vi "checkSamplingRates.vi"(8 "error in (no error)":errorcluster, 11 "Available Sigals in":refnum<class "ISignal.lvclass">[](array[class])) -> (0 "error out":errorcluster, 1 "SampleRate":dbl, 2 "Boolean":bool, 3 "Array":refnum<class "ISignal.lvclass">[](array[class]))   [LabVIEW 2022 SP3, in "MultiReader.lvlib"]
uses:
  <instrlib>/openDAQ/Examples/MultiReader/MultiReader.lvlib
  <instrlib>/openDAQ/Public/Classes/ISignal/ISignal.lvclass
  <instrlib>/openDAQ/Public/Classes/IBaseObject/Polymorphic/queryInterface/queryNumberInterface.vi
  <instrlib>/openDAQ/Public/Classes/IDataDescriptor/IDataDescriptor.lvclass
  <instrlib>/openDAQ/Public/Classes/IDataRule/IDataRule.lvclass
  <instrlib>/openDAQ/Public/Classes/daqCoreTypes/IRatio/IRatio.lvclass
  <instrlib>/openDAQ/Public/Classes/daqCoreTypes/IDict/IDict.lvclass
  <instrlib>/openDAQ/Public/Classes/IBaseObject/IBaseObject.lvclass
  <instrlib>/openDAQ/Public/Classes/daqCoreTypes/INumber/INumber.lvclass
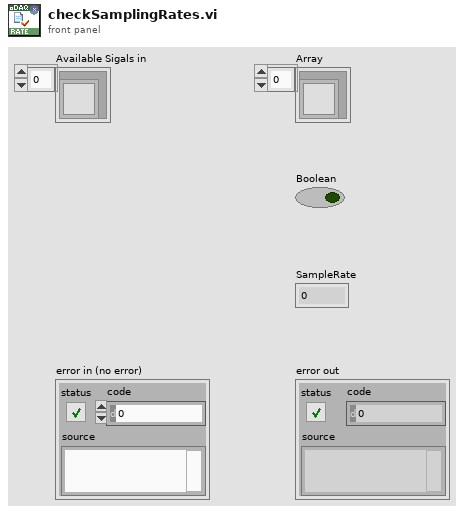
[diagram p1: front panel]
types:
  T1 = typedef "openDAQ.lvlib/IBaseObject.lvlib/IDataRule.lvlib/IDataRule.lvclass/DataRuleType.ctl" = u16
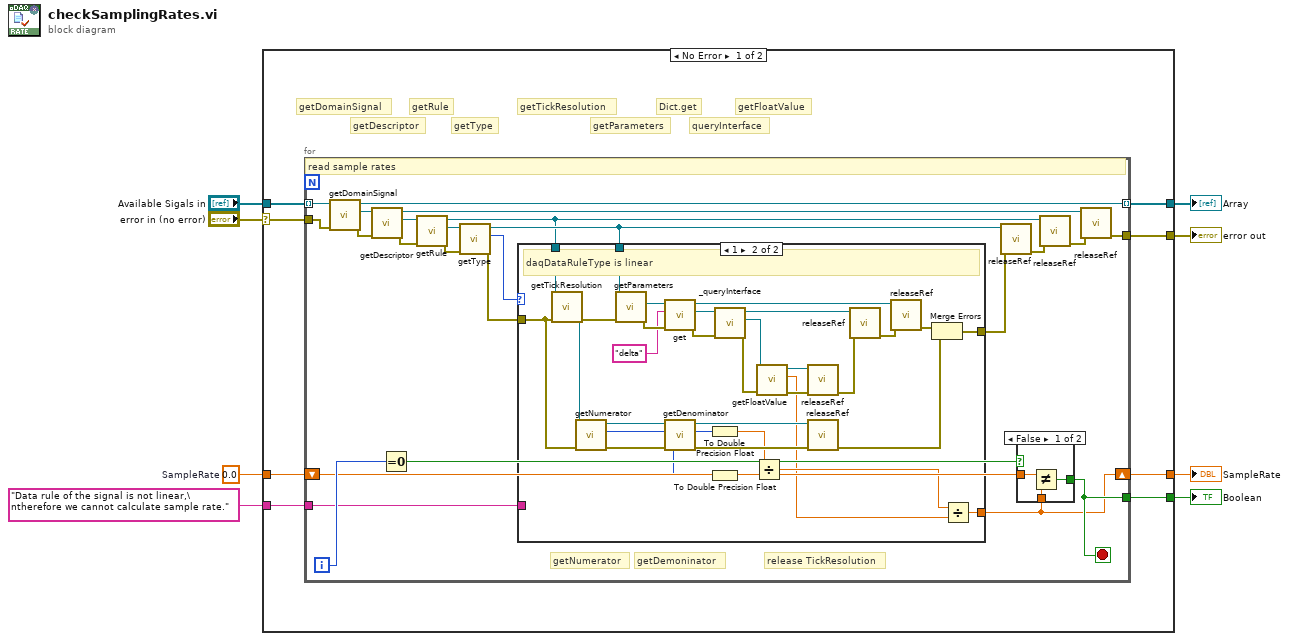
[diagram p0: block diagram]
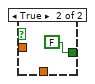
[diagram p2: hidden frame]
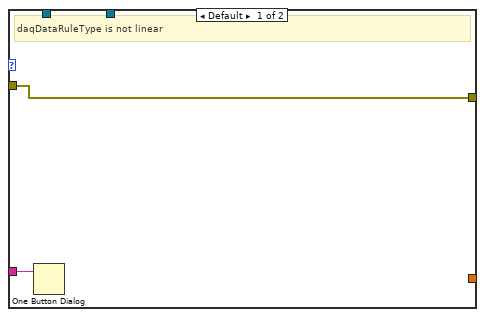
[diagram p3: hidden frame]
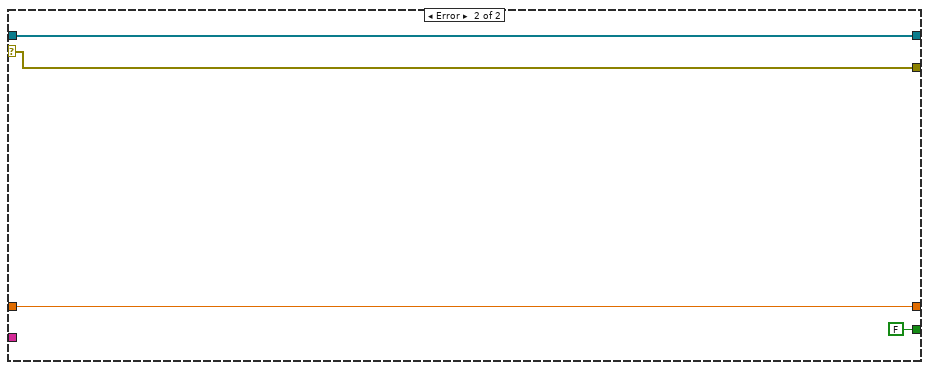
[diagram p4: hidden frame]
diagram:
  w3 = 0.0  # SampleRate
  n1 = case shown="No Error" "error in (no error)" {
    selector: "error in (no error)" -> [w9 w81]
    tunnel: [w16 w82] -> w8
    tunnel: [w15 w80] -> w7
    tunnel: "Data rule of the signal is not linear,\ntherefore we cannot calculate sample rate." ("modulePath") -> [w14 _]
    tunnel: [w13 FALSE] -> w5
    tunnel: [w12 w81] -> w4
    tunnel: w3 -> [w11 w80]
    tunnel: "Available Sigals in" -> [w10 w82]
    frame No Error {
      # "getFloatValue"
      # "queryInterface"
      # "Dict.get"
      # "getParameters"
      # "getTickResolution"
      # "getType"
      # "getRule"
      # "getDescriptor"
      # "getDomainSignal"
      n2 = for {
        tunnel: w10 -> [w22] mode=indexing
        tunnel: [w26] -> w12
        tunnel: w9 -> [w39]
        tunnel: w14 -> [w29]
        tunnel: [w21] -> w16 mode=indexing
        shift-right: [w18] -> w15
        shift-left: w11 -> [w20]
        tunnel: [w19] -> w13
        i -> [w40]
        stop <- w19 stop-if-true
        # "release TickResolution"
        # "getDemoninator"
        # "getNumerator"
        # "read sample rates"
        n3 = call <instrlib>:"getDomainSignal.vi"("error in (no error)"=w39, "ISignal in"=w22) -> ("error out"=w23:errorcluster, "DomainSignal out"=w38:refnum<class "ISignal.lvclass">, "ISignal out"=w21:refnum<class "ISignal.lvclass">)  [unwired: 7 in]
        n4 = call <instrlib>:"getDescriptor.vi"("error in (no error)"=w23, "ISignal in"=w38) -> ("error out"=w24:errorcluster, "DataDescriptor out"=w25:refnum<class "IDataDescriptor.lvclass">, "ISignal out"=w28:refnum<class "ISignal.lvclass">)  [unwired: 7 in]
        n5 = Equal To 0?(x=w40) -> (x = 0?=w17:bool)
        n6 = call <instrlib>:"getRule.vi"("error in (no error)"=w24, "IDataDescriptor in"=w25) -> ("error out"=w34:errorcluster, "DataRule out"=w35:refnum<class "IDataRule.lvclass">, "IDataDescriptor out"=w27:refnum<class "IDataDescriptor.lvclass">)  [unwired: 7 in]
        n7 = call <instrlib>:"getType.vi"("error in (no error)"=w34, "IDataRule in"=w35) -> ("error out"=w32:errorcluster, "DataRuleType"=w33:T1, "IDataRule out"=w31:refnum<class "IDataRule.lvclass">)  [unwired: 7 in]
        n8 = case shown="1" w33 {
          tunnel: w29 -> [w46 _]
          tunnel: w32 -> [w45 w63]
          tunnel: w27 -> [_ w75]
          tunnel: w31 -> [_ w73]
          tunnel: [w45 w54] -> w30
          tunnel: [_ w53] -> w18
          frame Default {
            # "daqDataRuleType is not linear"
            n9 = One Button Dialog(message=w46) -> ()  [unwired: 1 in, 1 out]
          }
          frame 1 {
            # "daqDataRuleType is linear"
            n10 = call <instrlib>:"getTickResolution.vi"("error in (no error)"=w63, "IDataDescriptor in"=w75) -> ("error out"=w74:errorcluster, "TickResolution out"=w65:refnum<class "IRatio.lvclass">)  [unwired: 7 in, 1 out]
            n11 = call <instrlib>:"getNumerator.vi"("error in (no error)"=w63, "IRatio in"=w65) -> ("error out"=w62:errorcluster, "Numerator out"=w59:i64, "IRatio out"=w64:refnum<class "IRatio.lvclass">)  [unwired: 7 in]
            n12 = call <instrlib>:"getParameters.vi"("error in (no error)"=w74, "IDataRule in"=w73) -> ("error out"=w52:errorcluster, "Parameters out"=w72:refnum<class "IDict.lvclass">)  [unwired: 7 in, 1 out]
            n13 = call <instrlib>:"get.vi"("error in (no error)"=w52, "Key in"="delta" ("String"), "IDict in"=w72) -> ("error out"=w49:errorcluster, "Value out"=w51:refnum<class "IBaseObject.lvclass">, "IDict out"=w57:refnum<class "IDict.lvclass">)  [unwired: 6 in]
            n14 = call <instrlib>:"getDenominator.vi"("error in (no error)"=w62, "IRatio in"=w64) -> ("error out"=w76:errorcluster, "Denominator out"=w61:i64, "IRatio out"=w77:refnum<class "IRatio.lvclass">)  [unwired: 7 in]
            n15 = To Double Precision Float(number=w61) -> (double precision float=w60:dbl)
            n16 = To Double Precision Float(number=w59) -> (double precision float=w58:dbl)
            n17 = call-poly <instrlib>:"_queryInterface.vi"("error in (no error)"=w49, "IBaseObject in"=w51) -> ("error out"=w71:errorcluster, "INumber out"=w67:refnum<class "INumber.lvclass">, "IBaseObject out"=w66:refnum<class "IBaseObject.lvclass">)  [unwired: 7 in]
            n18 = Divide(x=w60, y=w58) -> (x/y=w48:dbl)
            n19 = call <instrlib>:"getFloatValue.vi"("error in (no error)"=w71, "INumber in"=w67) -> ("error out"=w69:errorcluster, "Float Value out"=w47:dbl, "INumber out"=w70:refnum<class "INumber.lvclass">)  [unwired: 7 in]
            n20 = call-dynamic "releaseRef.vi"("error in (no error)"=w69, "IBaseObject in"=w70) -> ("error out"=w68:errorcluster)  [unwired: 9 in]
            n21 = call-dynamic "releaseRef.vi"("error in (no error)"=w76, "IBaseObject in"=w77) -> ("error out"=w78:errorcluster)  [unwired: 9 in]
            n22 = call-dynamic "releaseRef.vi"("error in (no error)"=w68, "IBaseObject in"=w66) -> ("error out"=w56:errorcluster)  [unwired: 9 in]
            n23 = call-dynamic "releaseRef.vi"("error in (no error)"=w56, "IBaseObject in"=w57) -> ("error out"=w55:errorcluster)  [unwired: 9 in]
            n24 = Merge Errors(w55, w78) -> (w54:errorcluster)
            n25 = Divide(x=w48, y=w47) -> (x/y=w53:dbl)
          }
        }
        n26 = call-dynamic "releaseRef.vi"("error in (no error)"=w30, "IBaseObject in"=w31) -> ("error out"=w36:errorcluster)  [unwired: 9 in]
        n27 = case shown="False" w17 {
          tunnel: w20 -> [w42 _]
          tunnel: [w43 FALSE] -> w19
          tunnel: w18 -> [w41 _]
          frame False {
            n28 = Not Equal?(x=w42, y=w41) -> (x != y?=w43:bool)
          }
          frame True {
          }
        }
        n29 = call-dynamic "releaseRef.vi"("error in (no error)"=w36, "IBaseObject in"=w27) -> ("error out"=w37:errorcluster)  [unwired: 9 in]
        n30 = call-dynamic "releaseRef.vi"("error in (no error)"=w37, "IBaseObject in"=w28) -> ("error out"=w26:errorcluster)  [unwired: 9 in]
      }
    }
    frame Error {
    }
  }
  "Array" <- w8
  "SampleRate" <- w7
  "Boolean" <- w5
  "error out" <- w4
